vi "read_exptime.vi"() -> ()   [LabVIEW 2020]
panel:
  out "lavgexp":i32
  out "error out":errorcluster caption="エラー出力"
  in  "error in":errorcluster caption="エラー入力"
  out "exp_sec":sgl
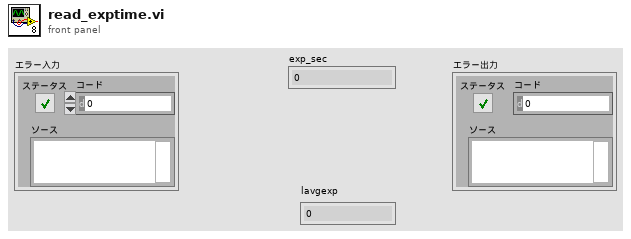
[diagram p1: front panel]
types:
  T1 = enum16{"open", "open or create", "create or replace", "create", "open (read only)"}
  T2 = enum16{"open", "replace", "create", "open or create", "replace or create", "replace or create with confirmation"}
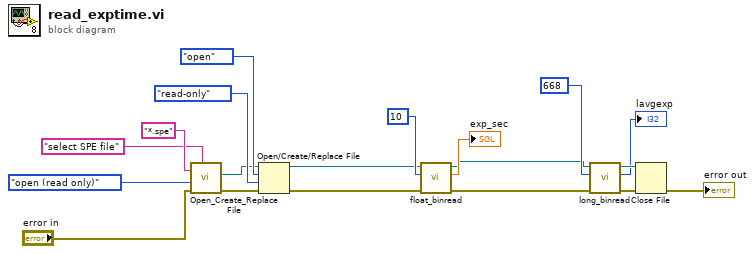
[diagram p0: block diagram]
diagram:
  n1 = call <vilib>:"Open_Create_Replace File.vi"("pattern"="*.spe", "prompt"="select SPE file", "error in (no error)"="error in", "function (open:0)"=T1."open (read only)") -> ("error out"=w15:errorcluster, "new file path"=w16:path)  [unwired: 4 in, 2 out]
  n2 = Open/Create/Replace File(file path (use dialog)=w16, error in=w15, operation (0:open)=T2."open", access (0:read/write)=enum16{"read/write", "read-only", "write-only"}."read-only" ("アクセス （0:read/write）")) -> (refnum out=w4:refnum<file>, error out=w3:errorcluster)  [unwired: 2 in, 1 out]
  n3 = call "float_binread.vi"("error in"=w3, "offset"=i64 10, "ref in"=w4) -> ("error out"=w2:errorcluster, "float"=→"exp_sec":sgl, "ref out"=w1:refnum<file>)  [unwired: 6 in]
  n4 = call "long_binread.vi"("error in"=w2, "offset"=i64 668, "ref in"=w1) -> ("error out"=w10:errorcluster, "long"=→"lavgexp":i32, "ref out"=w9:refnum<file>)  [unwired: 6 in]
  n5 = Close File(refnum=w9, error in=w10) -> (error out=→"error out":errorcluster)  [unwired: 1 out]
